vi "题目7.vi"() -> ()   [LabVIEW 2017]
uses:
  <vilib>/Utility/file.llb/Read Delimited Spreadsheet (DBL).vi
  <vilib>/Analysis/NI_AALBase.lvlib
panel:
  out "波形图表":dbl[][](graph)
  out "all rows":dbl[][](array[numeric]) caption="所有行"
  in  "cycles":dbl=1.0 caption="周期" format="%0.2f"
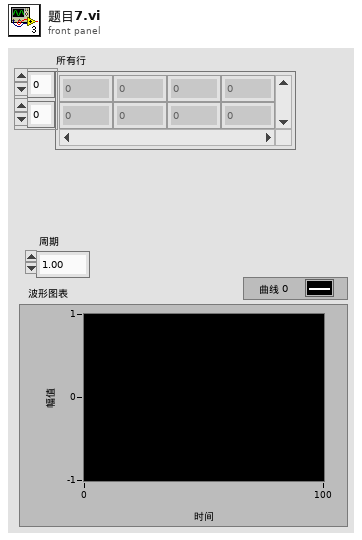
[diagram p1: front panel]
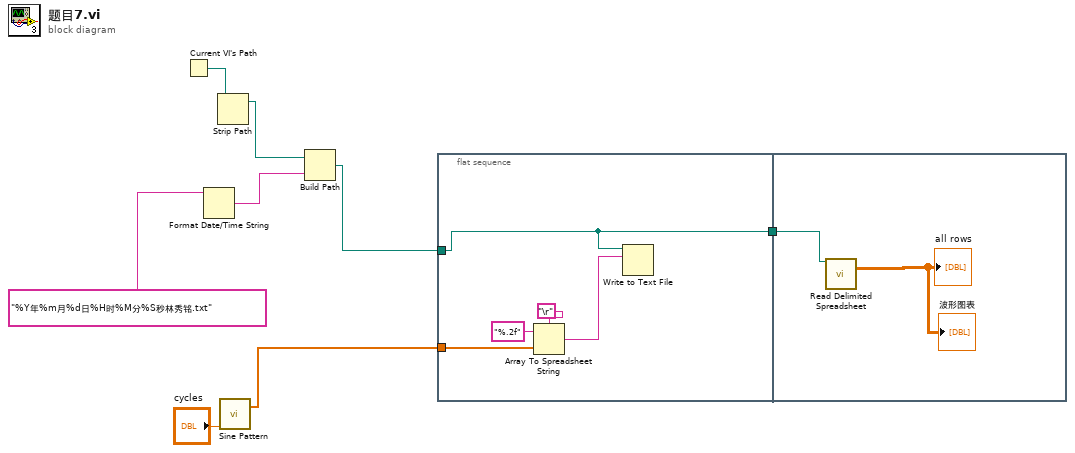
[diagram p0: block diagram]
diagram:
  n1 = Current VI's Path() -> (path=w8:path)
  n2 = Format Date/Time String(time format string (%c)="%Y年%m月%d日%H时%M分%S秒林秀铭.txt") -> (date/time string=w7:string)  [unwired: 2 in]
  n3 = Strip Path(path=w8) -> (stripped path=w6:path)  [unwired: 1 out]
  n4 = call <vilib>:"Sine Pattern.vi"("cycles"="cycles") -> ("Sinusoidal Pattern"=w2:dbl[])  [unwired: 3 in, 1 out]
  n5 = Build Path(base path=w6, name or relative path=w7) -> (appended path=w3:path)
  n6 = flat-sequence {
    tunnel: w3 -> [w9]
    tunnel: w2 -> [w13]
    tunnel: [w9] -> w1
    tunnel: w1 -> [w15]
    frame #0 {
      n7 = Array To Spreadsheet String(delimiter (Tab)="\r", array=w13, 3:"%.2f" ("格式字符串")) -> (spreadsheet string=w10:string)
      n8 = Write to Text File(file (use dialog)=w9, text=w10) -> ()  [unwired: 2 in, 3 out]
    }
    frame #1 {
      n9 = call-poly <vilib>:"Read Delimited Spreadsheet.vi"("file path (dialog if empty)"=w15) -> ("all rows"=→"all rows" →"波形图表":dbl[][])  [unwired: 9 in, 5 out]
    }
  }
